vi "Dashboard Main.vi"() -> ()   [LabVIEW 2012]
uses:
  NonDriveDisplayPanel.ctl
  Robot/util/Commands.ctl
  Robot/mecanum/mecanum_control.ctl
  Robot/Shooter/shooter_cmds.ctl
  Robot/climber/climber_cmds.ctl
  <vilib>/Utility/config.llb/Read Key (String).vi
  <vilib>/Utility/config.llb/Read Key (I32).vi
  <vilib>/Utility/config.llb/NI_LVConfig.lvlib
  <vilib>/vision/NI_Vision_Development_Module.lvlib
panel:
  out "Status":T1(ring)
  out "Mechanism Display":T2 {"Current Shooter VBus" scale=0.0..1.0; "Shooter Angle" scale=-10.0..40.0}
  in  "Running w/ Camera?":bool=TRUE
  out "Camera Image":T3(plugin-control)
  out "Master Caution":bool
  out "Battery Value":dbl(slide) scale=0.0..14.0 scale format="%#_2e"
  out "Battery":sgl(graph)
  out "Mode":T4(ring)=enum."Auto Disabled"
  out "Camera IP":string
  out "Robot IP":string
  # "Robot IP:"
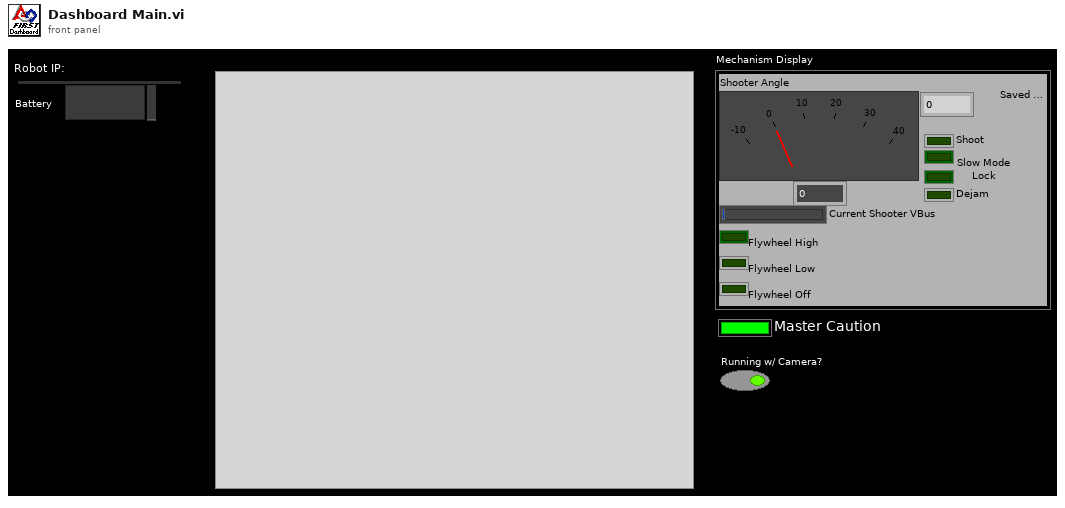
[diagram p1: front panel]
types:
  T1 = enum8{"Disconnected", "E-Stop", "Disabled", "Enabled"}
  T2 = typedef "NonDriveDisplayPanel.ctl" = cluster{"Shooter Angle":dbl, "Current Shooter VBus":dbl, "Flywheel High":bool, "Saved Angle":dbl, "Slow Mode":bool, "Lock":bool, "Flywheel Off ":bool, "Flywheel Low":bool, "Dejam":bool, "Shoot":bool}
  T3 = typedef "IMAQ Image.ctl" = refnum<image>
  T4 = enum8{"Tele-Op Disabled", "Tele-Op Enabled", "Auto Disabled", "Auto Enabled", "Test Disabled", "Test Enabled", ""}
  T5 = typedef "Image Type" = u32
  T6 = typedef "Commands.ctl" = cluster{"Mecanum":T7, "Shooter":T8, "Climber_Commands":T9}
  T7 = typedef "mecanum_control.ctl" = cluster{"Forward":dbl, "Strafe":dbl, "Rotate":dbl}
  T8 = typedef "shooter_cmds.ctl" = cluster{"Elevation":dbl, "Shoot":bool, "F_High":bool, "F_Low":bool, "F_Off":bool, "Slow_Mode":bool, "Lock":bool, "Dejam":bool}
  T9 = typedef "climber_cmds.ctl" = cluster{"Climber_Motor_Voltage":dbl}
  T10 = cluster{"Competition mode":bool, "Robot Link":bool, "Autonomous":bool, "Enabled":bool, "E-Stop":bool, "Simulated":bool, "TestMode":bool, "Docked Window":bool}
  T11 = typedef "LVRectTypeDef.ctl" = cluster{"Left":i16, "Top":i16, "Right":i16, "Bottom":i16}
  T12 = typedef "NI_LVConfig.lvlib/Config Data RefNum.ctl" = refnum<k1>
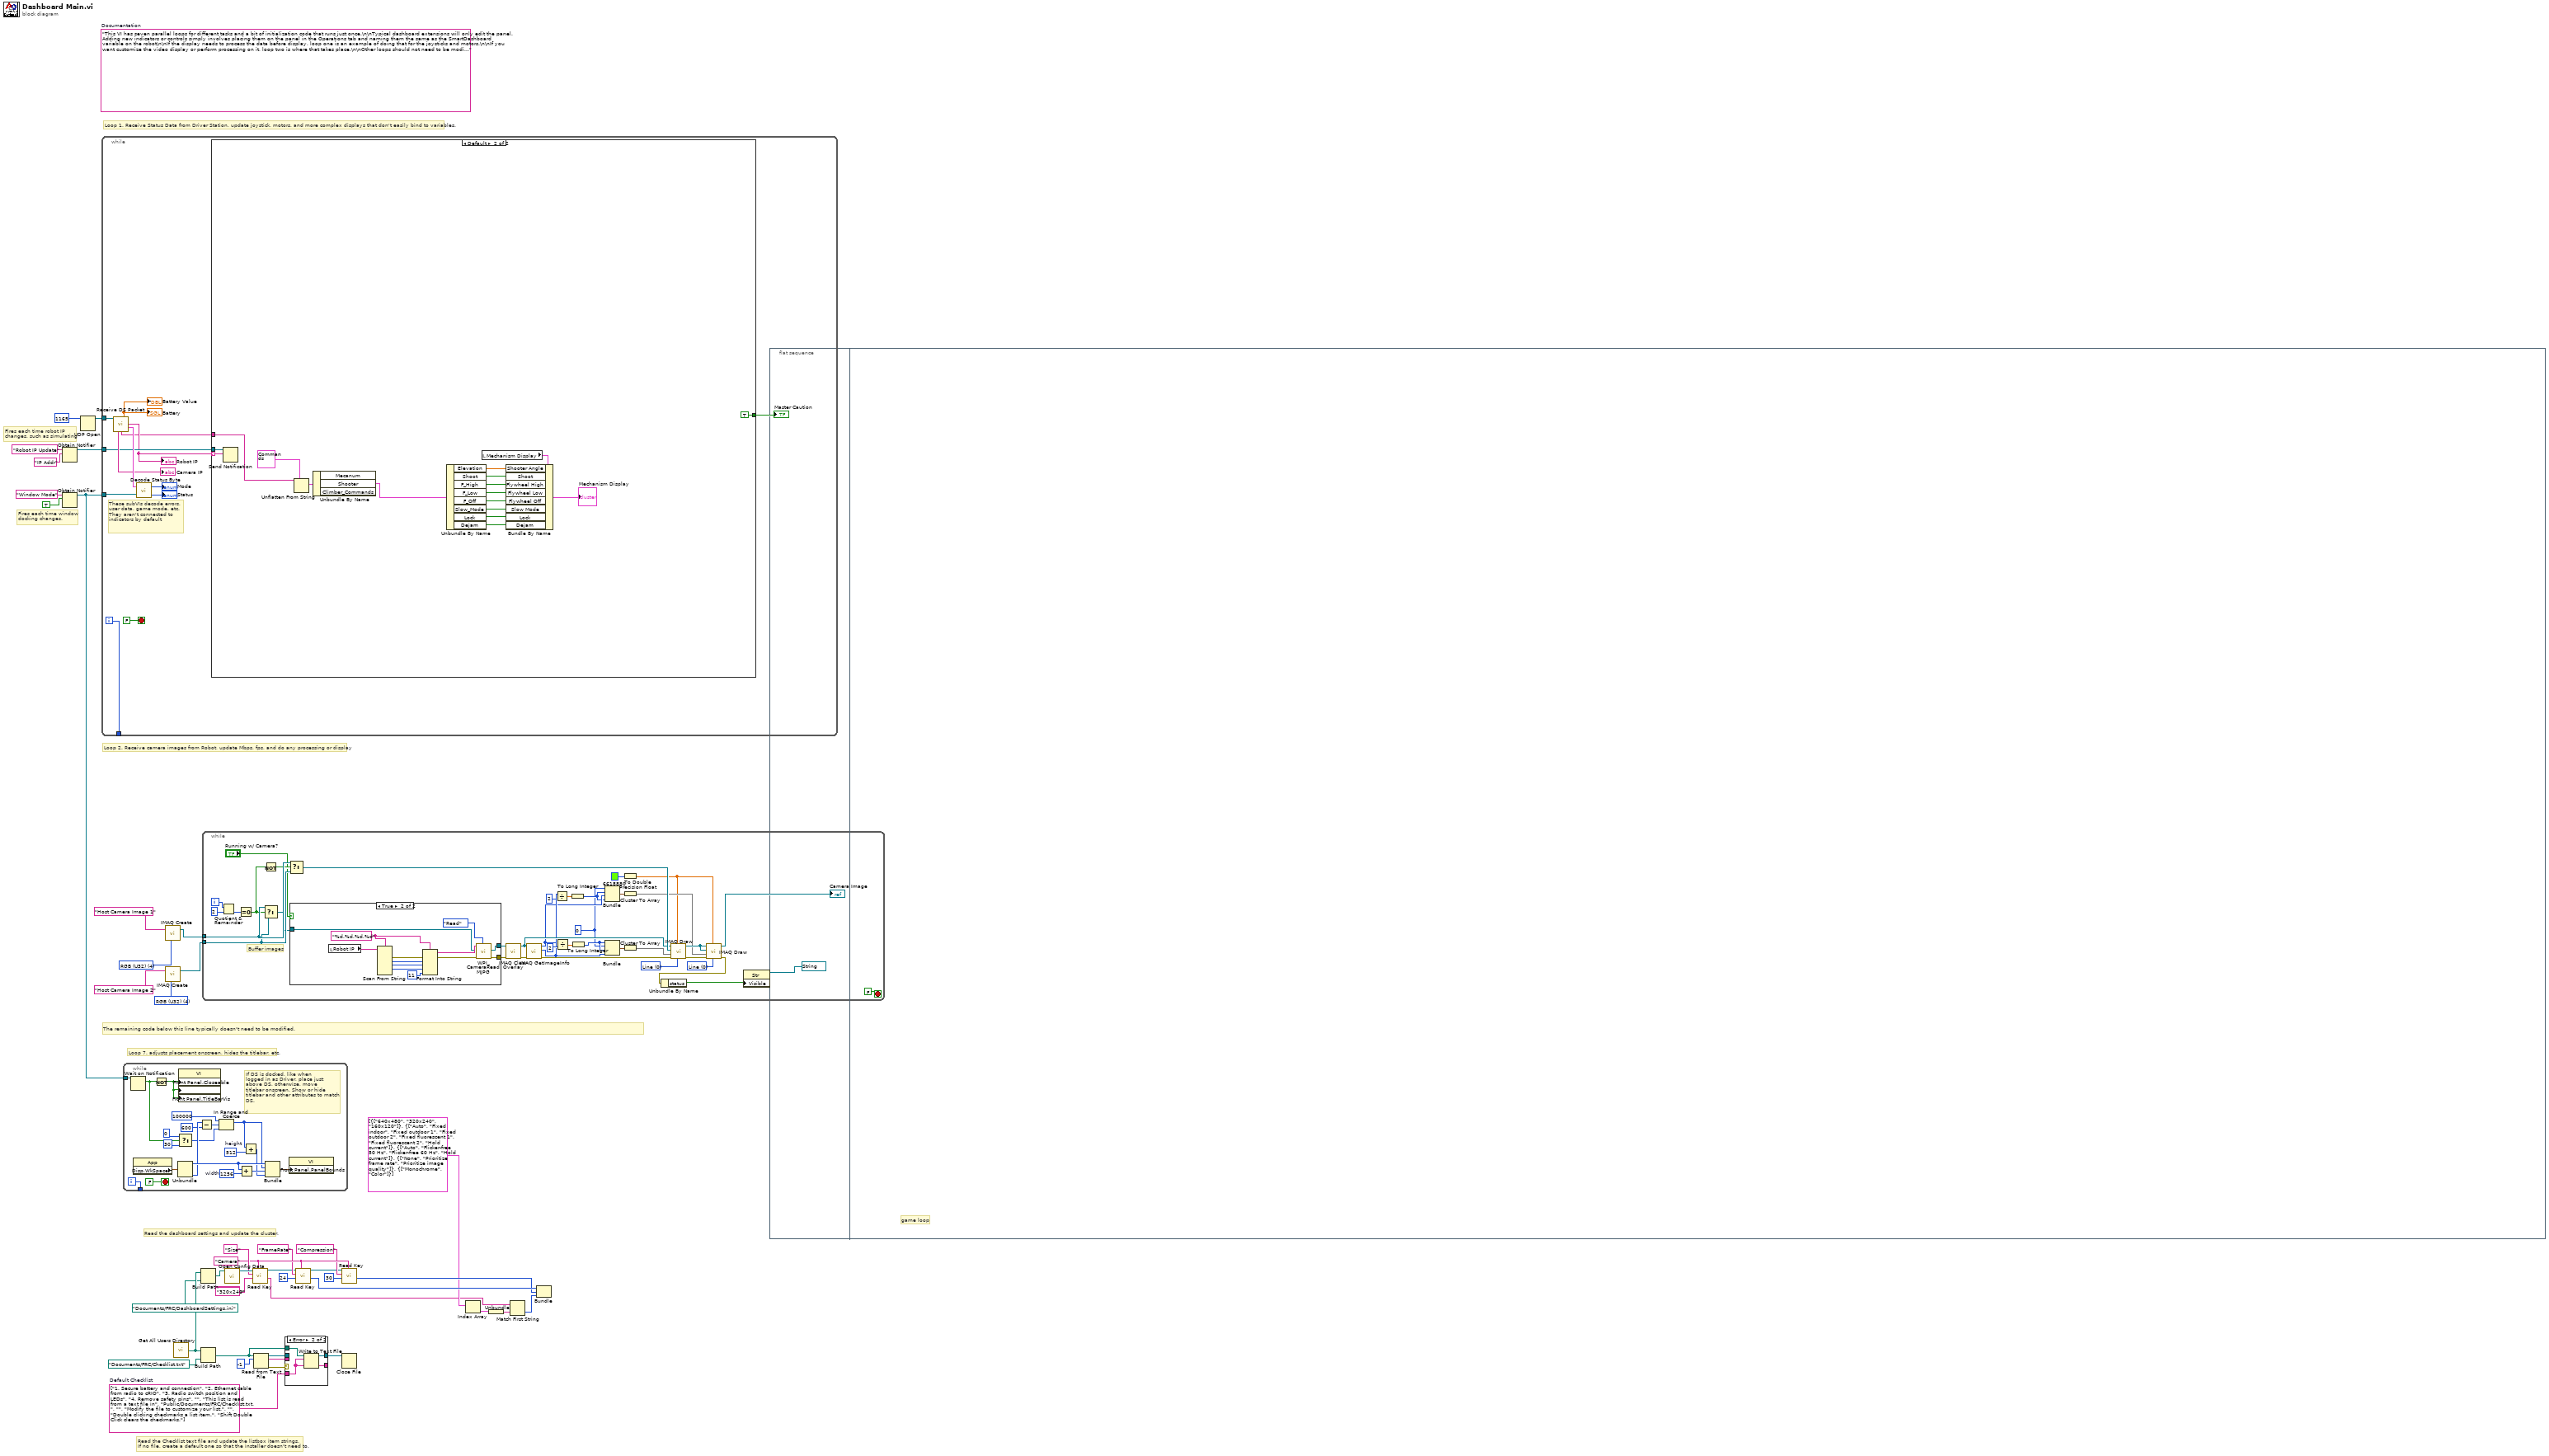
[diagram p0: block diagram]
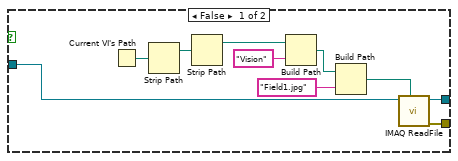
[diagram p2: hidden frame]
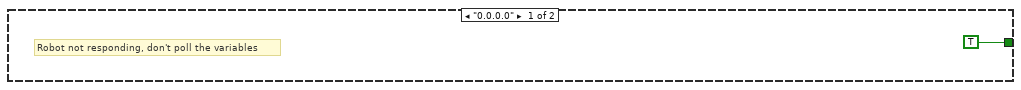
[diagram p4: hidden frame]
diagram:
  (unwired) "320x240"
  w3 = T5 4 items=["Grayscale (U8)", "Grayscale (I16)", "Grayscale (SGL)", "Complex (CSG)", "RGB (U32)", "HSL (U32)", "RGB (U64)", "Grayscale (U16)"] ("Image Type")
  w6 = T5 4 items=["Grayscale (U8)", "Grayscale (I16)", "Grayscale (SGL)", "Complex (CSG)", "RGB (U32)", "HSL (U32)", "RGB (U64)"] ("Image Type")
  w23 = "Camera"
  w29 = string[] ["1. Secure battery and connection", "2. Ethernet cable from radio to cRIO", "3. Radio switch position and LEDs", "4. Remove safety pins", "", "This list is read from a text file in", "Public/Documents/FRC/Checklist.txt.", "", "Modify the file to customize your list.", "", "Double clicking checkmarks a list item.", "Shift Double Click clears the checkmarks."]  # Default Checklist
  (unwired) "This VI has seven parallel loops for different tasks and a bit of initialization code that runs just once.\n\nTypical dashboard extensions will only edit the panel. Adding new indicators or controls simply involves placing them on the panel in the Operations tab and naming them the same as the SmartDashboard variable on the robot\n\nIf the display needs to process the data before display, loop one is an example of doing that for the joysticks and motors.\n\nIf you want customize the video display or perform processing on it, loop two is where that takes place.\n\nOther loops should not need to be modified. They are pretty standard, and document the task they perform."  # Documentation
  # "Fires each time robot IP\nchanges, such as simulating"
  # "Fires each time window\ndocking changes."
  # "Read the Checklist text file and update the listbox item strings.\nIf no file, create a default one so that the installer doesn't need to."
  # "The remaining code below this line typically doesn't need to be modified."
  # "Read the dashboard settings and update the cluster."
  # "Loop 7. adjusts placement onscreen, hides the titlebar, etc."
  # "Loop 1. Receive Status Data from Driver Station, update joystick, motors, and more complex displays that don't easily bind to variables."
  # "Loop 2. Receive camera images from Robot, update Mbps, fps, and do any processing or display"
  n1 = Obtain Notifier(name (unnamed)="Robot IP Update", notification data type="IP Addr" ("name (unnamed)")) -> (notifier out=w38:refnum<notifier>)  [unwired: 2 in, 2 out]
  n2 = Obtain Notifier(name (unnamed)="Window Mode", notification data type=TRUE) -> (notifier out=w33:refnum<notifier>)  [unwired: 2 in, 2 out]
  n3 = UDP Open(11:u16 1165 ("port")) -> (port=w41:refnum<k16>)  [unwired: 2 in, 4 out]
  n4 = while {
    tunnel: w41 -> [w53]
    tunnel: w38 -> [w47]
    tunnel: w33 -> [w51]
    tunnel: [w48] -> _
    i -> [w48]
    stop <- FALSE stop-if-true
    # "These subVIs decode errors, user data, game mode, etc.\nThey aren't connected to indicators by default"
    n5 = call "Receive DS Packet.vi"("Recv Socket"=w53) -> ("Battery"=→"Battery" →"Battery Value":sgl, "Robot IP Address"=w46:string, "Status"=w54:T10, "Camera IP Address"=→"Camera IP":string, "Low Priority User Data"=w43:string)  [unwired: 1 in, 9 out]
    "Robot IP" <- w46
    n6 = call "Decode Status Byte.vi"("Window Mode Notifier"=w51, "Status"=w54) -> ("Status"=→"Status":T1, "Mode"=→"Mode":T4)
    n7 = case shown="Default" w46 {
      selector: w46 -> [_ w72]
      tunnel: w47 -> [_ w73]
      tunnel: [TRUE TRUE] -> w45
      tunnel: w43 -> [_ w69]
      frame "0.0.0.0" {
        # "Robot not responding, don't poll the variables"
      }
      frame Default {
        n8 = Send Notification(notification=w72, notifier=w73) -> ()  [unwired: 1 in, 2 out]
        n9 = Unflatten From String(type=T6 {"Mecanum"={"Forward"=0.0, "Strafe"=0.0, "Rotate"=0.0}, "Shooter"={"Elevation"=0.0, "Shoot"=FALSE, "F_High"=FALSE, "F_Low"=FALSE, "F_Off"=FALSE, "Slow_Mode"=FALSE, "Lock"=FALSE, "Dejam"=FALSE}, "Climber_Commands"={"Climber_Motor_Voltage"=0.0}} ("Commands"), binary string=w69) -> (value=w68:T6)  [unwired: 3 in, 2 out]
        n10 = Unbundle By Name(w68) -> ("Shooter"=w67:T8)  [unwired: 2 out]
        n11 = Unbundle By Name(w67) -> ("Elevation"=w66:dbl, "Shoot"=w65:bool, "F_High"=w64:bool, "F_Low"=w63:bool, "F_Off"=w62:bool, "Slow_Mode"=w61:bool, "Lock"=w60:bool, "Dejam"=w59:bool)
        n12 = local read "Mechanism Display"() -> (w70:T2)
        n13 = Bundle By Name(cluster=w70, "Shooter Angle"=w66, "Shoot"=w65, "Flywheel High"=w64, "Flywheel Low"=w63, "Flywheel Off"=w62, "Slow Mode"=w61, "Lock"=w60, "Dejam"=w59) -> (→"Mechanism Display":T2)
      }
    }
    "Master Caution" <- w45
  }
  n14 = while {
    tunnel: w33 -> [w92]
    tunnel: [w90] -> _
    i -> [w90]
    stop <- FALSE stop-if-true
    w82 = 1256  # width
    w85 = 512  # height
    # "If DS is docked, like when\nlogged in as Driver, place just\nabove DS, otherwise, move\ntitlebar onscreen. Show or hide\ntitlebar and other attributes to match\nDS."
    n15 = Wait on Notification(notifier=w92) -> (notification=w77:bool)  [unwired: 3 in, 3 out]
    n16 = property class="App"() -> ("Disp.WkSpace"=w88:T11)  [unwired: 2 in, 2 out]
    n17 = Not(x=w77) -> (.not. x?=w91:bool)
    n18 = Unbundle(w88) -> ("Left"=w86:i16, "Bottom"=w83:i16)  [unwired: 2 out]
    n19 = Select(t=0, s=w77, f=30) -> (s? t:f=w76:i32)
    n20 = property class="VI"("Front Panel.Closeable"=w91, "Front Panel.Minimizeable"=w91, "Front Panel.TitleBarVis"=w91) -> ()  [unwired: 2 in, 2 out]
    n21 = Subtract(x=w83, y=600) -> (x-y=w80:i32)
    n22 = In Range and Coerce(upper limit=100000, x=w80, lower limit=w76) -> (coerced(x)=w74:i32)  [unwired: 1 out]
    n23 = Add(x=w86, y=w82) -> (x+y=w87:i32)
    n24 = Add(x=w74, y=w85) -> (x+y=w84:i32)
    n25 = Bundle("Left"=w86, w74, w87, w84) -> (w89:cluster{"Left":i16, i32, i32, i32})  [unwired: 1 out]
    n26 = property class="VI"("Front Panel.PanelBounds"=w89) -> ()  [unwired: 2 in, 2 out]
  }
  n27 = call "IMAQ Create"("Image Name"="Host Camera Image 1", "Image Type"=w6) -> ("New Image"=w2:T3)  [unwired: 2 in, 2 out]
  n28 = call "IMAQ Create"("Image Name"="Host Camera Image 2", "Image Type"=w3) -> ("New Image"=w1:T3)  [unwired: 3 in, 1 out]
  n29 = call "Get All Users Directory.vi"() -> ("All User Path"=w28:path)
  n30 = Build Path(base path=w28, name or relative path=path "Documents/FRC/DashboardSettings.ini") -> (appended path=w27:path)
  n31 = Build Path(base path=w28, name or relative path=path "Documents/FRC/Checklist.txt") -> (appended path=w30:path)
  n32 = while {
    tunnel: w2 -> [w131]
    tunnel: w1 -> [w126]
    i -> [w130]
    stop <- FALSE stop-if-true
    w105 = u16 0 items=["Line", "Rectangle", "Oval"] ("Shape to draw")
    w97 = 0
    w125 = u16 0 items=["Line", "Rectangle", "Oval"] ("Shape to draw")
    # "Buffer images"
    n33 = Quotient & Remainder(x=w130, y=2) -> (floor(x/y)=w128:i32)  [unwired: 1 out]
    n34 = Equal To 0?(x=w128) -> (x = 0?=w127:bool)
    n35 = Not(x=w127) -> (.not. x?=w116:bool)
    n36 = Select(t=w131, s=w127, f=w126) -> (s? t:f=w113:T3)
    n37 = Select(t=w131, s=w116, f=w126) -> (s? t:f=w115:T3)
    n38 = case shown="True" "Running w/ Camera?" {
      tunnel: w113 -> [w142 w145]
      tunnel: [w140 w143] -> w118
      tunnel: [w141 w144] -> w117
      frame False {
        n39 = Current VI's Path() -> (path=w139:path)
        n40 = Strip Path(path=w139) -> (stripped path=w138:path)  [unwired: 1 out]
        n41 = Strip Path(path=w138) -> (stripped path=w133:path)  [unwired: 1 out]
        n42 = Build Path(base path=w133, name or relative path="Vision") -> (appended path=w136:path)
        n43 = Build Path(base path=w136, name or relative path="Field1.jpg") -> (appended path=w134:path)
        n44 = call "IMAQ ReadFile"("File Path"=w134, "Image"=w142) -> ("error out"=w140:errorcluster, "Image Out"=w141:T3)  [unwired: 5 in, 3 out]
      }
      frame True {
        w149 = "%d.%d.%d.%d" ("format string")
        n45 = local read "Robot IP"() -> (w146:string)
        n46 = Scan From String(format string=w149, input string=w146) -> (error out=w152:errorcluster, output 1=w153:i32, output 2=w154:i32, output 3=w155:i32)  [unwired: 2 in, 7 out]
        n47 = Format Into String(format string=w149, error in=w152, w153, w154, w155, 11 ("IP Suffix:")) -> (resulting string=w151:string, error out=w150:errorcluster)  [unwired: 1 in]
        n48 = call <vilib>:"WPI_CameraRead MJPG.vi"("Operation"=enum16{"Read", "Reopen", "Close"}."Read", "error in"=w150, "Image"=w145, "address"=w151) -> ("error out"=w143:errorcluster, "Image Out"=w144:T3)  [unwired: 5 in, 1 out]
      }
    }
    n49 = call "IMAQ Clear Overlay"("error in (no error)"=w118, "Image"=w117) -> ("error out"=w111:errorcluster, "Image Out"=w112:T3)  [unwired: 8 in]
    n50 = call "IMAQ GetImageInfo"("error in (no error)"=w111, "Image"=w112) -> ("error out"=w119:errorcluster, "Y Resolution"=w102:i32, "X Resolution"=w99:i32)  [unwired: 2 in, 5 out]
    n51 = Divide(x=w102, y=2) -> (x/y=w100:dbl)
    n52 = Divide(x=w99, y=2) -> (x/y=w123:dbl)
    n53 = To Long Integer(number=w100) -> (32bit integer=w98:i32)
    n54 = To Long Integer(number=w123) -> (32bit integer=w122:i32)
    n55 = Bundle(w97, w98, "X Resolution"=w99, w98) -> (w104:cluster{i32, i32, "X Resolution":i32, i32})  [unwired: 1 in]
    n56 = Bundle(w122, w97, w122, "Y Resolution"=w102) -> (w121:cluster{i32, i32, i32, "Y Resolution":i32})  [unwired: 1 in]
    n57 = Cluster To Array(cluster=w104) -> (array=w103:i32[])
    n58 = Cluster To Array(cluster=w121) -> (array=w120:i32[])
    n59 = To Double Precision Float(number=u32 6618880) -> (double precision float=w95:dbl)
    n60 = call "IMAQ Draw"("Shape to draw"=w125, "Pixel Color"=w95, "error in (no error)"=w119, "Coordinates"=w120, "Image Dst"=w115, "Image Src"=w112) -> ("error out"=w108:errorcluster, "Image Dst Out"=w106:T3)  [unwired: 4 in]
    n61 = call "IMAQ Draw"("Shape to draw"=w105, "Pixel Color"=w95, "error in (no error)"=w108, "Coordinates"=w103, "Image Dst"=w106, "Image Src"=w106) -> ("error out"=w107:errorcluster, "Image Dst Out"=→"Camera Image":T3)  [unwired: 4 in]
    n62 = Unbundle By Name(w107) -> ("status"=w110:bool)
    n63 = property on="Property Node" class="Str"(reference=refnum<vi> refnum, "Visible"=w110) -> ()  [unwired: 1 in, 2 out]
  }
  n64 = call <vilib>:"Open Config Data.vi"("configuration file path"=w27) -> ("refnum"=w26:T12)  [unwired: 8 in, 2 out]
  n65 = call-poly <vilib>:"Read Key.vi"("section"=w23, "default value"="320x240", "key"="Size", "refnum"=w26) -> ("value"=w13:string, "refnum out"=w8:T12)  [unwired: 2 in, 4 out]
  n66 = Read from Text File(file (use dialog)=w30, count=-1 ("timeout ms (25000)")) -> (refnum out=w10:refnum<file>, text=w31:string[], error out=w32:errorcluster)  [unwired: 2 in, 1 out]
  n67 = case shown="Error" w32 {
    tunnel: w31 -> [w157 _]
    tunnel: [w157 w159] -> _
    tunnel: w29 -> [_ w159]
    tunnel: w30 -> [_ w160]
    tunnel: [w156 w158] -> w9
    tunnel: w10 -> [w156 _]
    frame No Error {
    }
    frame Error {
      n68 = Write to Text File(file (use dialog)=w160, text=w159) -> (refnum out=w158:refnum<file>)  [unwired: 2 in, 2 out]
    }
  }
  n69 = call-poly <vilib>:"Read Key.vi"("section"=w23, "default value"=24, "key"="FrameRate", "refnum"=w8) -> ("value"=w18:i32, "refnum out"=w7:T12)  [unwired: 1 in, 5 out]
  n70 = Close File(refnum=w9) -> ()  [unwired: 1 in, 2 out]
  n71 = call-poly <vilib>:"Read Key.vi"("section"=w23, "default value"=30, "key"="Compression", "refnum"=w7) -> ("value"=w17:i32)  [unwired: 1 in, 6 out]
  n72 = Index Array(array=cluster{string[]}[] [{["640x480", "320x240", "160x120"]}, {["Auto", "Fixed indoor", "Fixed outdoor 1", "Fixed outdoor 2", "Fixed fluorescent 1", "Fixed fluorescent 2", "Hold current"]}, {["Auto", "Flicker-free 50 Hz", "Flicker-free 60 Hz", "Hold current"]}, {["None", "Prioritize frame rate", "Prioritize image quality"]}, {["Monochrome", "Color"]}]) -> (element=w16:cluster{string[]})  [unwired: 1 in]
  n73 = Unbundle(w16) -> (w14:string[])
  n74 = Match First String(2:w14, 3:w13) -> (0:w12:i32)  [unwired: 1 out]
  n75 = Bundle("value"=w18, "value"=w17, "index"=w12) -> ()  [unwired: 2 out]
  n76 = flat-sequence {
    frame #0 {
    }
    frame #1 {
      # "game loop"
    }
  }
